vi "Reverse 2D Array__ogtk.vi"   [LabVIEW 2014]
doc: "This polymorphic VI reverses the input 2D <B>Array</B> and outputs the result as <B>Reversed Array</B>. Use the <B>by rows or columns</B> input to specify whether to sort by row or by column."
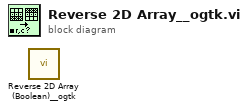
[diagram p0: block diagram]
diagram:
  n1 = call "Reverse 2D Array (Boolean)__ogtk.vi"() -> ()  [unwired: 3 in, 1 out]
